vi "voltage divider.vi"() -> ()   [LabVIEW 2019]
panel:
  in  "Vs":dbl(slide) scale=0.0..100.0
  out "V2":dbl(knob) scale=0.0..100.0
  in  "R2":dbl
  in  "R1":dbl
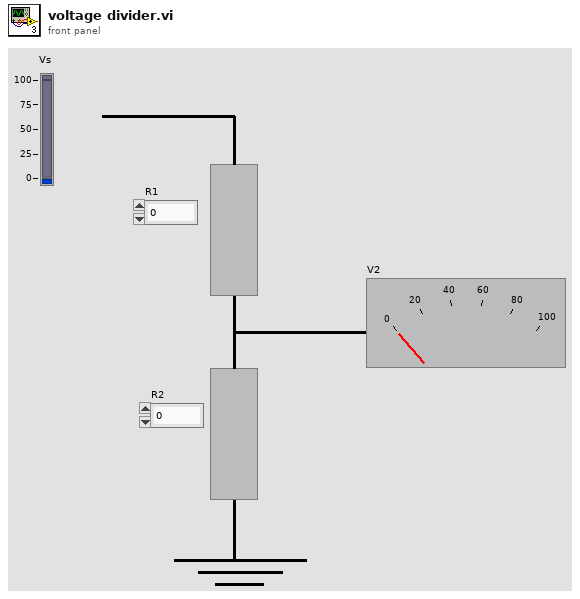
[diagram p1: front panel]
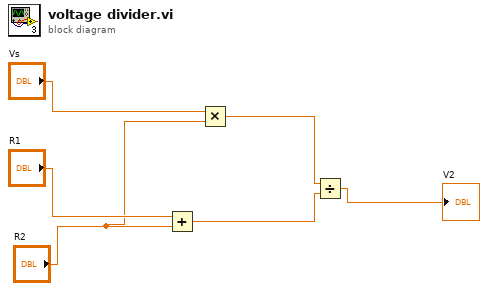
[diagram p0: block diagram]
diagram:
  n1 = Add(x="R1", y="R2") -> (x+y=w2:dbl)
  n2 = Multiply(x="Vs", y="R2") -> (x*y=w3:dbl)
  n3 = Divide(x=w3, y=w2) -> (x/y=→"V2":dbl)
